vi "VGA_pulso.vi"(7 "Espera acceso USB":u32=10, 8 "error in":errorcluster, 9 "Frecuencia pulso (0.2 a 1 Mhz)":dbl=1000000.0 format="%0_2p", 10 "Patrón (E000)":u16=57344 format="%04x", 11 "ftHandle_in":u32) -> (0 "error out":errorcluster, 3 "ftHandle_out":u32)   [LabVIEW 2019]
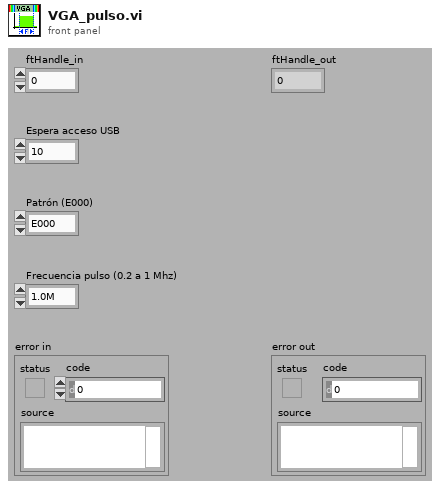
[diagram p1: front panel]
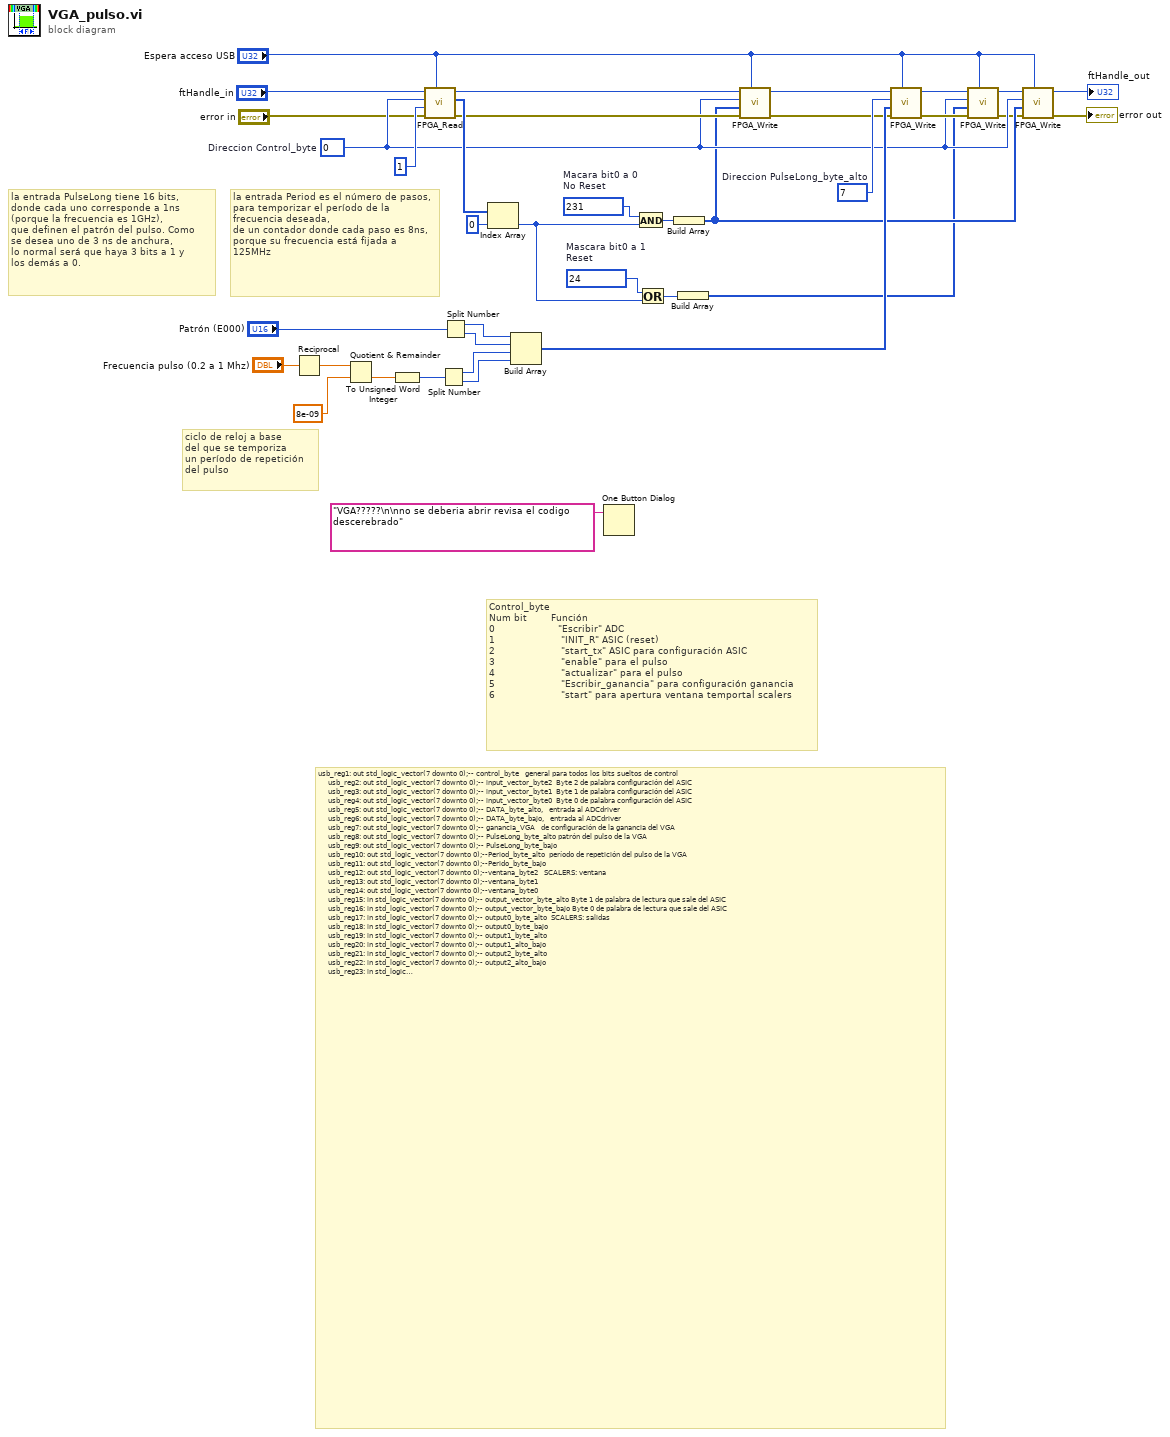
[diagram p0: block diagram]
diagram:
  w34 = u8 7  # Direccion PulseLong_byte_alto
  w29 = u8 24  # Mascara bit0 a 1 Reset
  w27 = u8 231  # Macara bit0 a 0 No Reset
  w19 = u8 0  # Direccion Control_byte
  # "la entrada Period es el número de pasos, para temporizar el período de la frecuencia deseada,\nde un contador donde cada paso es 8ns, porque su frecuencia está fijada a 125MHz"
  # "la entrada PulseLong tiene 16 bits,\ndonde cada uno corresponde a 1ns \n(porque la frecuencia es 1GHz), \nque definen el patrón del pulso. Como\nse desea uno de 3 ns de anchura, \nlo normal será que haya 3 bits a 1 y \nlos demás a 0."
  # "Control_byte\nNum bit        Función\n0                     \"Escribir\" ADC\n1                      \"INIT_R\" ASIC (reset)\n2                      \"start_tx\" ASIC para configuración ASIC\n3                      \"enable\" para el pulso\n4                      \"actualizar\" para el pulso\n5                      \"Escribir_ganancia\" para configuración ganancia\n6                      \"start\" para apertura ventana temportal scalers"
  # "usb_reg1: out std_logic_vector(7 downto 0);-- control_byte\t\t\tgeneral para todos los bits sueltos de control\n\t\t\t  usb_reg2: out std_logic_vector(7 downto 0);-- input_vector_byte2 \tByte 2 de palabra configuración del ASIC\n\t\t\t  usb_reg3: out std_logic_vector(7 downto 0);-- input_vector_byte1 \tByte 1 de palabra configuración del ASIC\n\t\t\t  usb_reg4: out std_logic_vector(7 downto 0);-- input_vector_byte0 \tByte 0 de palabra configuración del ASIC\n\t\t\t  usb_reg5: out std_logic_vector(7 downto 0);-- DATA_byte_alto, \t\tentrada al ADCdriver\n\t\t\t  usb_reg6: out std_logic_vector(7 downto 0);-- DATA_byte_bajo, \t\tentrada al ADCdriver\n\t\t\t  usb_reg7: out std_logic_vector(7 downto 0);-- ganancia_VGA\t\t\tde configuración de la ganancia del VGA\n\t\t\t  usb_reg8: out std_logic_vector(7 downto 0);-- PulseLong_byte_alto\tpatrón del pulso de la VGA\n\t\t\t  usb_reg9: out std_logic_vector(7 downto 0);-- PulseLong_byte_bajo\n\t\t\t  usb_reg10: out std_logic_vector(7 downto 0);--Period_byte_alto\t\tperíodo de repetición del pulso de la VGA\n\t\t\t  usb_reg11: out std_logic_vector(7 downto 0);--Perido_byte_bajo\n\t\t\t  usb_reg12: out std_logic_vector(7 downto 0);--ventana_byte2\t\t\tSCALERS: ventana\n\t\t\t  usb_reg13: out std_logic_vector(7 downto 0);--ventana_byte1\t\n\t\t\t  usb_reg14: out std_logic_vector(7 downto 0);--ventana_byte0\n\t\t\t  usb_reg15: in std_logic_vector(7 downto 0);-- output_vector_byte_alto\tByte 1 de palabra de lectura que sale del ASIC\n\t\t\t  usb_reg16: in std_logic_vector(7 downto 0);-- output_vector_byte_bajo\tByte 0 de palabra de lectura que sale del ASIC\n\t\t\t  usb_reg17: in std_logic_vector(7 downto 0);-- output0_byte_alto\t\tSCALERS: salidas\n\t\t\t  usb_reg18: in std_logic_vector(7 downto 0);-- output0_byte_bajo\n\t\t\t  usb_reg19: in std_logic_vector(7 downto 0);-- output1_byte_alto\n\t\t\t  usb_reg20: in std_logic_vector(7 downto 0);-- output1_alto_bajo \n\t\t\t  usb_reg21: in std_logic_vector(7 downto 0);-- output2_byte_alto \n\t\t\t  usb_reg22: in std_logic_vector(7 downto 0);-- output2_alto_bajo \n\t\t\t  usb_reg23: in std_logic_vector(7 downto 0);-- para el canal_0 del ADCdriver\n\t\t\t  usb_reg24: in std_logic_vector(7 downto 0);\n\t\t\t  usb_reg25: in std_logic_vector(7 downto 0);-- para el canal_1 del ADCdriver\n\t\t\t  usb_reg26: in std_logic_vector(7 downto 0);\n\t\t\t  usb_reg27: in std_logic_vector(7 downto 0);-- para el canal_2 del ADCdriver\n\t\t\t  usb_reg28: in std_logic_vector(7 downto 0);\n\t\t\t  usb_reg29: in std_logic_vector(7 downto 0);-- para el canal_3 del ADCdriver\n\t\t\t  usb_reg30: in std_logic_vector(7 downto 0);\n\t\t\t  usb_reg31: in std_logic_vector(7 downto 0);-- para el canal_4 del ADCdriver\n\t\t\t  usb_reg32: in std_logic_vector(7 downto 0);\n\t\t\t  usb_reg33: in std_logic_vector(7 downto 0);-- para el canal_5 del ADCdriver\n\t\t\t  usb_reg34: in std_logic_vector(7 downto 0);\n\t\t\t  usb_reg35: in std_logic_vector(7 downto 0);-- para el canal_6 del ADCdriver\n\t\t\t  usb_reg36: in std_logic_vector(7 downto 0);\n\t\t\t  usb_reg37: in std_logic_vector(7 downto 0);-- para el canal_7 del ADCdriver\n\t\t\t  usb_reg38: in std_logic_vector(7 downto 0);\n\t\t\t  usb_reg39: in std_logic_vector(7 downto 0);-- para el canal_8 del ADCdriver\n\t\t\t  usb_reg40: in std_logic_vector(7 downto 0);\n\t\t\t  usb_reg41: in std_logic_vector(7 downto 0);-- para el canal_9 del ADCdriver\n\t\t\t  usb_reg42: in std_logic_vector(7 downto 0);\n\t\t\t  usb_reg43: in std_logic_vector(7 downto 0);-- para el canal_10 del ADCdriver\n\t\t\t  usb_reg44: in std_logic_vector(7 downto 0)--;"
  # "ciclo de reloj a base\ndel que se temporiza\nun período de repetición\ndel pulso"
  n1 = Reciprocal(x="Frecuencia pulso (0.2 a 1 Mhz)") -> (1/x=w13:dbl)
  n2 = Quotient & Remainder(x=w13, y=8e-09 ("x")) -> (floor(x/y)=w11:dbl)  [unwired: 1 out]
  n3 = To Unsigned Word Integer(number=w11) -> (unsigned 16bit integer=w10:u16)
  n4 = call "FPGA_Read.vi"("Espera acceso USB"="Espera acceso USB", "error in"="error in", "Numero Bytes"=u8 1, "Dirección base"=w19, "ftHandle_in"="ftHandle_in") -> ("error out"=w22:errorcluster, "lpBuffer_out"=w23:u8[], "ftHandle_out"=w21:u32)  [unwired: 2 in, 2 out]
  n5 = Split Number(x=w10) -> (hi(x)=w9:u8, lo(x)=w8:u8)
  n6 = Split Number(x="Patrón (E000)") -> (hi(x)=w35:u8, lo(x)=w36:u8)
  n7 = Index Array(array=w23, index=0) -> (element=w28:u8)
  n8 = Build Array(w35, w36, w9, w8) -> (w37:u8[])
  n9 = One Button Dialog(message="VGA?????\n\nno se deberia abrir revisa el codigo descerebrado") -> ()  [unwired: 1 in, 1 out]
  n10 = And(x=w27, y=w28) -> (x .and. y?=w25:u8)
  n11 = Or(x=w29, y=w28) -> (x .or. y?=w26:u8)
  n12 = Build Array(w25) -> (w18:u8[])
  n13 = Build Array(w26) -> (w15:u8[])
  n14 = call "FPGA_Write.vi"("Espera acceso USB"="Espera acceso USB", "error in"=w22, "Bytes de escritura"=w18, "Dirección base"=w19, "ftHandle_in"=w21) -> ("error out"=w31:errorcluster, "ftHandle_out"=w30:u32)  [unwired: 1 in, 2 out]
  n15 = call "FPGA_Write.vi"("Espera acceso USB"="Espera acceso USB", "error in"=w31, "Bytes de escritura"=w37, "Dirección base"=w34, "ftHandle_in"=w30) -> ("error out"=w33:errorcluster, "ftHandle_out"=w32:u32)  [unwired: 1 in, 2 out]
  n16 = call "FPGA_Write.vi"("Espera acceso USB"="Espera acceso USB", "error in"=w33, "Bytes de escritura"=w15, "Dirección base"=w19, "ftHandle_in"=w32) -> ("error out"=w16:errorcluster, "ftHandle_out"=w17:u32)  [unwired: 1 in, 2 out]
  n17 = call "FPGA_Write.vi"("Espera acceso USB"="Espera acceso USB", "error in"=w16, "Bytes de escritura"=w18, "Dirección base"=w19, "ftHandle_in"=w17) -> ("error out"=→"error out":errorcluster, "ftHandle_out"=→"ftHandle_out":u32)  [unwired: 1 in, 2 out]
